vi "Frame History Process.vi"(8 "error in (no error)":errorcluster, 11 "Video Processor in":refnum<class "Video Processor.lvclass">) -> (0 "error out":errorcluster, 2 "Depth Values Out":dbl[](array[numeric]), 3 "Video Processor out":refnum<class "Video Processor.lvclass">)   [LabVIEW 2018, in "Video Processor.lvclass"]
uses:
  Video Processor.lvclass
  C:/Users/aaron.jencks/Documents/GitHub/emerson_seed_object_detection/LabVIEW/Projects/Paul's Video Viewer/Classes/Video File/Video File.lvclass
  Video Processor.lvclass/Video Processor.ctl
  ROIed Video Frame/ROIed Video Frame.lvclass
  c87be4e5-8fdf-42f6-9462-9481252edd96.vi
  bee54c7f-775e-4ed8-afa5-e4368d0ff3cb.vi
  8f7f2294-6759-4051-832e-ebf1a1c5e352.vi
  <vilib>/Analysis/baseanly.llb/Mean (DBL).vi
  8f7f2294-6759-4051-832e-ebf1a1c5e352.vi/11446a4e-aecb-4e77-900c-abbc11fdc7f5.vi
  <vilib>/Analysis/NI_AALBase.lvlib
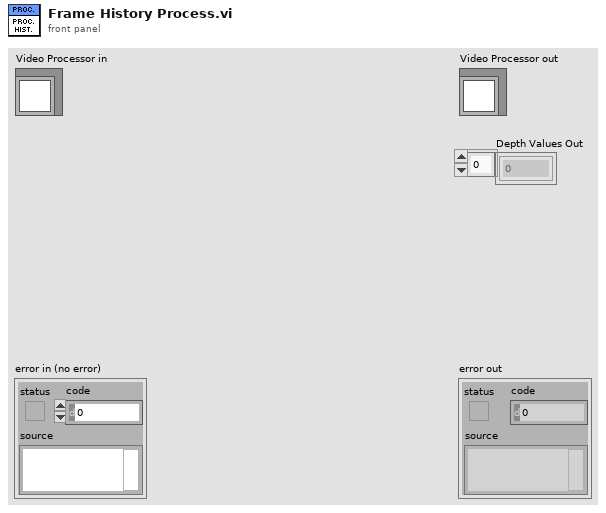
[diagram p1: front panel]
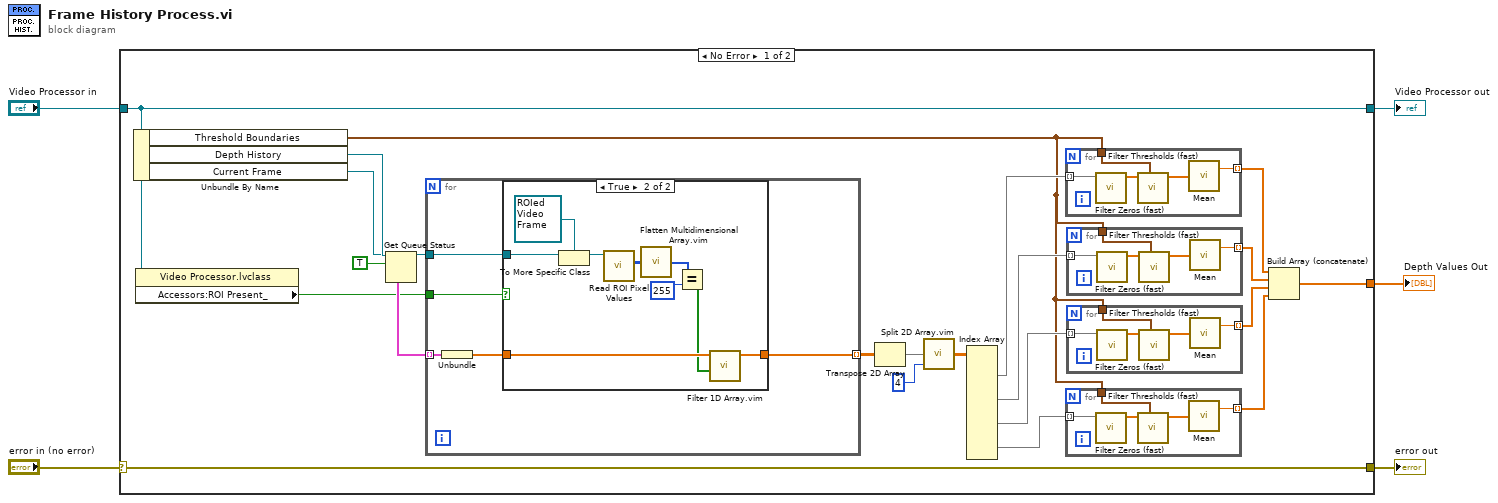
[diagram p0: block diagram]
diagram:
  n1 = case shown="No Error" "error in (no error)" {
    selector: "error in (no error)" -> [w19 w63]
    tunnel: [w19 w63] -> w1
    tunnel: [w22 w62] -> w3
    tunnel: "Video Processor in" -> [w22 w62]
    tunnel: [w10 _] -> w2
    frame No Error {
      n2 = Unbundle By Name(w22) -> ("Threshold Boundaries"=w11:cluster{"Minimum":dbl, "Maximum":dbl}, "Depth History"=w26:refnum<queue>, "Current Frame"=w23:refnum<class "Video Frame.lvclass">)
      n3 = property class="Video Processor.lvclass"(reference=w22) -> ("Accessors:ROI Present_"=w21:bool)  [unwired: 1 in, 2 out]
      n4 = Get Queue Status(queue=w26, return elements? (F)=TRUE) -> (elements=w24:cluster{"Array":dbl[]}[])  [unwired: 1 in, 7 out]
      n5 = for {
        tunnel: w24 -> [w51] mode=indexing
        tunnel: w23 -> [w50]
        tunnel: [w47] -> w20 mode=indexing
        tunnel: w21 -> [w48]
        n6 = Unbundle(w51) -> ("Array"=w49:dbl[])
        n7 = case shown="True" w48 {
          tunnel: w50 -> [_ w54]
          tunnel: w49 -> [w52 w58]
          tunnel: [w52 w56] -> w47
          frame False {
          }
          frame True {
            n8 = To More Specific Class(target class=refnum<class "ROIed Video Frame.lvclass"> refnum ("ROIed Video Frame.lvclass"), reference=w54) -> (specific class reference=w55:refnum<class "ROIed Video Frame.lvclass">)  [unwired: 1 in, 1 out]
            n9 = call-dynamic "Read ROI Pixel Values.vi"("ROIed Video Frame in"=w55) -> ("ROI Pixel Values"=w61:u8[][])  [unwired: 8 in, 2 out]
            n10 = call "Flatten Multidimensional Array.vim"("Array"=w61) -> ("output array"=w60:u8[])  [unwired: 14 in]
            n11 = Equal?(x=w60, y=u8 255) -> (x = y?=w57:bool[])
            n12 = call "Filter 1D Array.vim"("Boolean Filter"=w57, "Array"=w58) -> ("Array Out"=w56:dbl[])  [unwired: 9 in]
          }
        }
      }
      n13 = Transpose 2D Array(2D array=w20) -> (transposed array=w18:dbl[][])
      n14 = call "Split 2D Array.vim"("Number of segments (2)"=4, "Array"=w18) -> ("Split Array"=w16:dbl[][][])  [unwired: 1 in]
      n15 = Index Array(array=w16) -> (element #1=w15:dbl[][], element #2=w14:dbl[][], element #3=w13:dbl[][], element #4=w12:dbl[][])  [unwired: 12 in]
      n16 = for {
        tunnel: w15 -> [w30] mode=indexing
        tunnel: w11 -> [w27]
        tunnel: [w31] -> w9 mode=indexing
        n17 = call "Filter Zeros (fast).vi"("Array in"=w30) -> ("Array out"=w29:dbl[])  [unwired: 10 in]
        n18 = call "Filter Thresholds (fast).vi"("Thresholds"=w27, "Sorted Array"=w29) -> ("Filtered Array"=w28:dbl[])  [unwired: 9 in]
        n19 = call-poly <vilib>:"Mean.vi"("X"=w28) -> ("mean"=w31:dbl)  [unwired: 1 out]
      }
      n20 = for {
        tunnel: w12 -> [w35] mode=indexing
        tunnel: w11 -> [w33]
        tunnel: [w36] -> w6 mode=indexing
        n21 = call "Filter Zeros (fast).vi"("Array in"=w35) -> ("Array out"=w34:dbl[])  [unwired: 10 in]
        n22 = call "Filter Thresholds (fast).vi"("Thresholds"=w33, "Sorted Array"=w34) -> ("Filtered Array"=w32:dbl[])  [unwired: 9 in]
        n23 = call-poly <vilib>:"Mean.vi"("X"=w32) -> ("mean"=w36:dbl)  [unwired: 1 out]
      }
      n24 = for {
        tunnel: w14 -> [w40] mode=indexing
        tunnel: w11 -> [w38]
        tunnel: [w41] -> w8 mode=indexing
        n25 = call "Filter Zeros (fast).vi"("Array in"=w40) -> ("Array out"=w39:dbl[])  [unwired: 10 in]
        n26 = call "Filter Thresholds (fast).vi"("Thresholds"=w38, "Sorted Array"=w39) -> ("Filtered Array"=w37:dbl[])  [unwired: 9 in]
        n27 = call-poly <vilib>:"Mean.vi"("X"=w37) -> ("mean"=w41:dbl)  [unwired: 1 out]
      }
      n28 = for {
        tunnel: w13 -> [w45] mode=indexing
        tunnel: w11 -> [w43]
        tunnel: [w46] -> w7 mode=indexing
        n29 = call "Filter Zeros (fast).vi"("Array in"=w45) -> ("Array out"=w44:dbl[])  [unwired: 10 in]
        n30 = call "Filter Thresholds (fast).vi"("Thresholds"=w43, "Sorted Array"=w44) -> ("Filtered Array"=w42:dbl[])  [unwired: 9 in]
        n31 = call-poly <vilib>:"Mean.vi"("X"=w42) -> ("mean"=w46:dbl)  [unwired: 1 out]
      }
      n32 = Build Array (concatenate)(w9, w8, w7, w6) -> (w10:dbl[])
    }
    frame Error {
    }
  }
  "error out" <- w1
  "Video Processor out" <- w3
  "Depth Values Out" <- w2
